vi "PathPlanner_TrajectoryState25_Interpolate.vi"(9 "Time":dbl, 10 "end Val":T1={"TimeSeconds"=0.0, "LinearVelocity"=0.0, "Heading"={"VALUE"=0.0, "COS"=1.0, "SIN"=0.0}, "Constraints"={"MaxVelocityMps;"=0.0, "MaxAccelerationMpsSq;"=0.0, "MaxAngularVelRadPsEc;"=0.0, "MaxAngularAccRadPSecSq"=0.0, "Exists"=FALSE, "Unlimited"=FALSE, "NominalVoltageVolts"=12.0}, "DeltaPos"=0.0, "FieldSpeeds"={"vX"=0.0, "vY"=0.0, "vOmega"=0.0}, "pose"={"TRANSLATION"={"X"=0.0, "Y"=0.0}, "ROTATION"={"VALUE"=0.0, "COS"=1.0, "SIN"=0.0}}, "DeltaRot"={"VALUE"=0.0, "COS"=1.0, "SIN"=0.0}, "ModuleStates"=[], "WaypointRelPos"=0.0, "Feedforwards"={"accelerationsMPSSq"=[], "linearForcesNewtons"=[], "torqueCurrentsAmps"=[], "robotRelativeForcesXNewtons"=[], "robotRelativeForcesYNewtons"=[]}} {"ModuleStates"."SWERVE_DRIVE_MODULE_STATE"."Angle"."SIN" format="%13.4f"; "ModuleStates"."SWERVE_DRIVE_MODULE_STATE"."Angle"."COS" format="%13.4f"; "ModuleStates"."SWERVE_DRIVE_MODULE_STATE"."Angle"."VALUE" format="%13.4f"; "ModuleStates"."FieldAngle"."SIN" format="%13.4f"; "ModuleStates"."FieldAngle"."COS" format="%13.4f"; "ModuleStates"."FieldAngle"."VALUE" format="%13.4f"; "ModuleStates"."FieldPos"."Y" format="%14.3f"; "ModuleStates"."FieldPos"."X" format="%14.3f"; "DeltaRot"."SIN" format="%13.4f"; "DeltaRot"."COS" format="%13.4f"; "DeltaRot"."VALUE" format="%13.4f"; "pose"."ROTATION"."SIN" format="%13.4f"; "pose"."ROTATION"."COS" format="%13.4f"; "pose"."ROTATION"."VALUE" format="%13.4f"; "pose"."TRANSLATION"."Y" format="%14.3f"; "pose"."TRANSLATION"."X" format="%14.3f"; "FieldSpeeds"."vOmega" format="%10.3f"; "FieldSpeeds"."vY" format="%10.3f"; "FieldSpeeds"."vX" format="%10.3f"; "Heading"."SIN" format="%13.4f"; "Heading"."COS" format="%13.4f"; "Heading"."VALUE" format="%13.4f"}, 11 "in PathPlannerState":T1={"TimeSeconds"=0.0, "LinearVelocity"=0.0, "Heading"={"VALUE"=0.0, "COS"=1.0, "SIN"=0.0}, "Constraints"={"MaxVelocityMps;"=0.0, "MaxAccelerationMpsSq;"=0.0, "MaxAngularVelRadPsEc;"=0.0, "MaxAngularAccRadPSecSq"=0.0, "Exists"=FALSE, "Unlimited"=FALSE, "NominalVoltageVolts"=12.0}, "DeltaPos"=0.0, "FieldSpeeds"={"vX"=0.0, "vY"=0.0, "vOmega"=0.0}, "pose"={"TRANSLATION"={"X"=0.0, "Y"=0.0}, "ROTATION"={"VALUE"=0.0, "COS"=1.0, "SIN"=0.0}}, "DeltaRot"={"VALUE"=0.0, "COS"=1.0, "SIN"=0.0}, "ModuleStates"=[], "WaypointRelPos"=0.0, "Feedforwards"={"accelerationsMPSSq"=[], "linearForcesNewtons"=[], "torqueCurrentsAmps"=[], "robotRelativeForcesXNewtons"=[], "robotRelativeForcesYNewtons"=[]}} {"ModuleStates"."SWERVE_DRIVE_MODULE_STATE"."Angle"."SIN" format="%13.4f"; "ModuleStates"."SWERVE_DRIVE_MODULE_STATE"."Angle"."COS" format="%13.4f"; "ModuleStates"."SWERVE_DRIVE_MODULE_STATE"."Angle"."VALUE" format="%13.4f"; "ModuleStates"."FieldAngle"."SIN" format="%13.4f"; "ModuleStates"."FieldAngle"."COS" format="%13.4f"; "ModuleStates"."FieldAngle"."VALUE" format="%13.4f"; "ModuleStates"."FieldPos"."Y" format="%14.3f"; "ModuleStates"."FieldPos"."X" format="%14.3f"; "DeltaRot"."SIN" format="%13.4f"; "DeltaRot"."COS" format="%13.4f"; "DeltaRot"."VALUE" format="%13.4f"; "pose"."ROTATION"."SIN" format="%13.4f"; "pose"."ROTATION"."COS" format="%13.4f"; "pose"."ROTATION"."VALUE" format="%13.4f"; "pose"."TRANSLATION"."Y" format="%14.3f"; "pose"."TRANSLATION"."X" format="%14.3f"; "FieldSpeeds"."vOmega" format="%10.3f"; "FieldSpeeds"."vY" format="%10.3f"; "FieldSpeeds"."vX" format="%10.3f"; "Heading"."SIN" format="%13.4f"; "Heading"."COS" format="%13.4f"; "Heading"."VALUE" format="%13.4f"}) -> (3 "interpolated PathPlanner State":T1={"TimeSeconds"=0.0, "LinearVelocity"=0.0, "Heading"={"VALUE"=0.0, "COS"=1.0, "SIN"=0.0}, "Constraints"={"MaxVelocityMps;"=0.0, "MaxAccelerationMpsSq;"=0.0, "MaxAngularVelRadPsEc;"=0.0, "MaxAngularAccRadPSecSq"=0.0, "Exists"=FALSE, "Unlimited"=FALSE, "NominalVoltageVolts"=12.0}, "DeltaPos"=0.0, "FieldSpeeds"={"vX"=0.0, "vY"=0.0, "vOmega"=0.0}, "pose"={"TRANSLATION"={"X"=0.0, "Y"=0.0}, "ROTATION"={"VALUE"=0.0, "COS"=1.0, "SIN"=0.0}}, "DeltaRot"={"VALUE"=0.0, "COS"=1.0, "SIN"=0.0}, "ModuleStates"=[], "WaypointRelPos"=0.0, "Feedforwards"={"accelerationsMPSSq"=[], "linearForcesNewtons"=[], "torqueCurrentsAmps"=[], "robotRelativeForcesXNewtons"=[], "robotRelativeForcesYNewtons"=[]}} {"ModuleStates"."SWERVE_DRIVE_MODULE_STATE"."Angle"."SIN" format="%13.4f"; "ModuleStates"."SWERVE_DRIVE_MODULE_STATE"."Angle"."COS" format="%13.4f"; "ModuleStates"."SWERVE_DRIVE_MODULE_STATE"."Angle"."VALUE" format="%13.4f"; "ModuleStates"."FieldAngle"."SIN" format="%13.4f"; "ModuleStates"."FieldAngle"."COS" format="%13.4f"; "ModuleStates"."FieldAngle"."VALUE" format="%13.4f"; "ModuleStates"."FieldPos"."Y" format="%14.3f"; "ModuleStates"."FieldPos"."X" format="%14.3f"; "DeltaRot"."SIN" format="%13.4f"; "DeltaRot"."COS" format="%13.4f"; "DeltaRot"."VALUE" format="%13.4f"; "pose"."ROTATION"."SIN" format="%13.4f"; "pose"."ROTATION"."COS" format="%13.4f"; "pose"."ROTATION"."VALUE" format="%13.4f"; "pose"."TRANSLATION"."Y" format="%14.3f"; "pose"."TRANSLATION"."X" format="%14.3f"; "FieldSpeeds"."vOmega" format="%10.3f"; "FieldSpeeds"."vY" format="%10.3f"; "FieldSpeeds"."vX" format="%10.3f"; "Heading"."SIN" format="%13.4f"; "Heading"."COS" format="%13.4f"; "Heading"."VALUE" format="%13.4f"})   [LabVIEW 2019, in "PathPlanner24.lvlib"]
doc: "Interpolate between this state and the given state\n \nInputs: \n - trajectoryState - cluster - this trajectory state\n - endVal - cluster - State to interpolate with\n - t - double - Interpolation factor (0.0-1.0)\n\nOutputs:\n - Interpolated state - trajectory state - interpolated state"
uses:
  PathPlanner24.lvlib
  TypeDef/PathPlannerTrajectoryState25.ctl
  <vilib>/Rock Robotics/WPI/ThirdParty/JAS_Junk/TrajLib/TypeDef/ROTATION2D.ctl
  TypeDef/PathPlannerPathConstraints.ctl
  <vilib>/Rock Robotics/WPI/ThirdParty/JAS_Junk/TrajLib/TypeDef/CHASSIS_SPEEDS.ctl
  <vilib>/Rock Robotics/WPI/ThirdParty/JAS_Junk/TrajLib/TypeDef/POSE2D.ctl
  <vilib>/Rock Robotics/WPI/ThirdParty/JAS_Junk/TrajLib/TypeDef/TRANSLATION2D.ctl
  TypeDef/PathPlannerSwerveModTrajState.ctl
  <vilib>/Rock Robotics/WPI/ThirdParty/JAS_Junk/TrajLib/TypeDef/SWERVE_DRIVE_MODULE_STATE.ctl
  TypeDef/PathPlannerDriveFeedFwds.ctl
  <vilib>/Rock Robotics/WPI/ThirdParty/JAS_Junk/TrajLib/MathUtil_Interpolate.vi
  <vilib>/Rock Robotics/WPI/ThirdParty/JAS_Junk/TrajLib/Rotation2d_Minus.vi
  <vilib>/Rock Robotics/WPI/ThirdParty/JAS_Junk/TrajLib/Rotation2d_Times.vi
  <vilib>/Rock Robotics/WPI/ThirdParty/JAS_Junk/TrajLib/Rotation2d_Plus.vi
  <vilib>/Rock Robotics/WPI/ThirdParty/JAS_Junk/TrajLib/MathUtil_Clamp.vi
  <vilib>/Rock Robotics/WPI/ThirdParty/JAS_Junk/TrajLib/Rotation2d_UnaryMinus.vi
  <vilib>/Rock Robotics/WPI/ThirdParty/JAS_Junk/TrajLib/Rotation2d_RotateBy.vi
  <vilib>/Rock Robotics/WPI/ThirdParty/JAS_Junk/TrajLib/Rotation2d_CreateAngle.vi
  <vilib>/Rock Robotics/WPI/ThirdParty/JAS_Junk/TrajLib/Rotation2d_CreateXY.vi
  <vilib>/Rock Robotics/WPI/ThirdParty/JAS_Junk/TrajLib/Util_CalcDist.vi
  <vilib>/Rock Robotics/WPI/ThirdParty/JAS_Junk/TrajLib/Trajectory_Library.lvlib
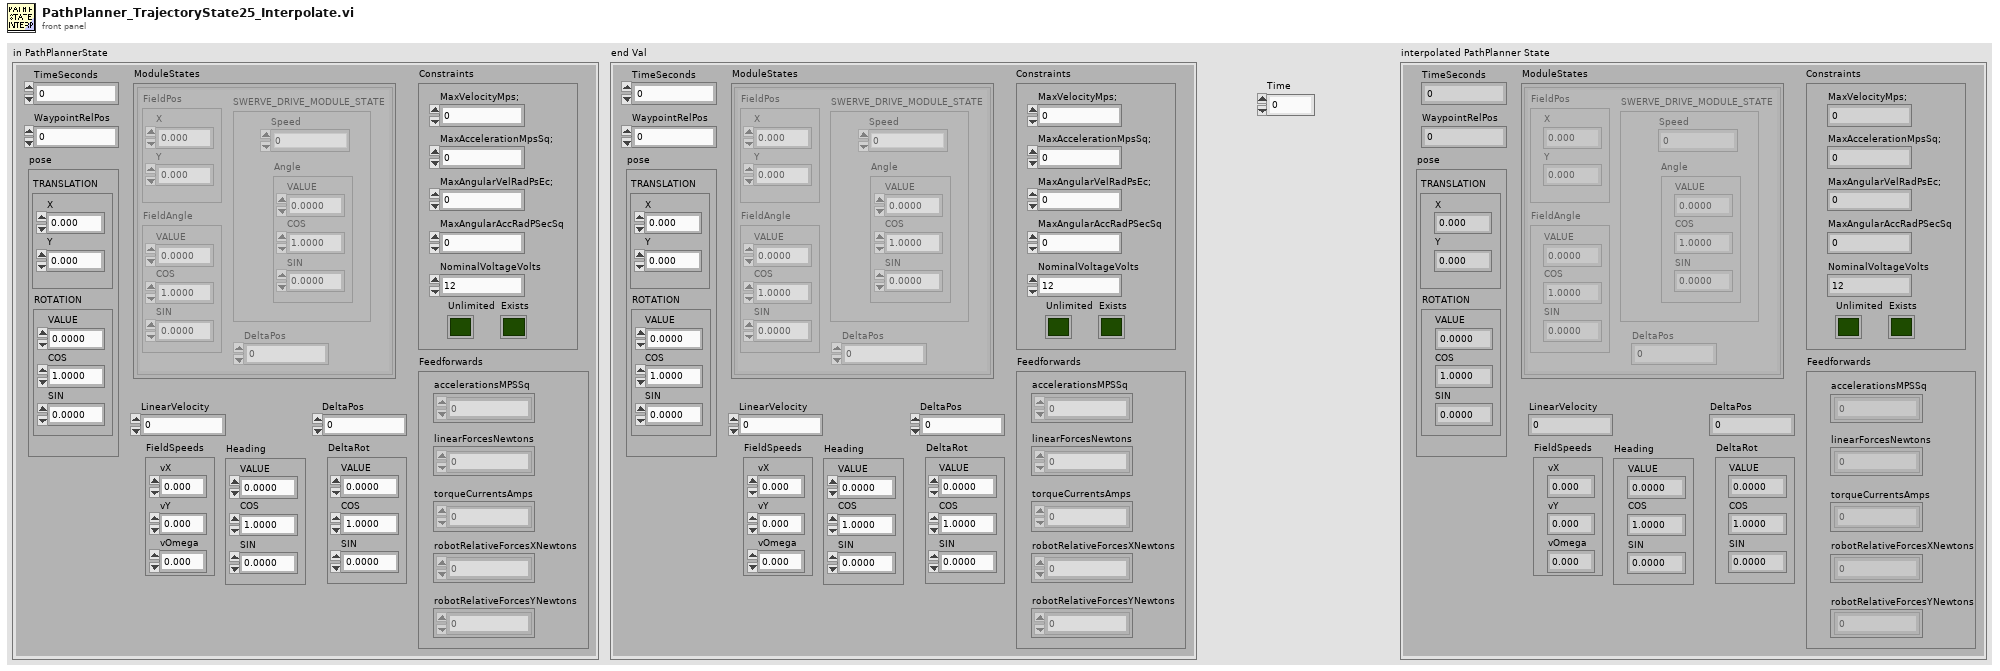
[diagram p1: front panel]
types:
  T1 = typedef "PathPlanner24.lvlib/PathPlannerTrajectoryState25.ctl" = cluster{"TimeSeconds":dbl, "LinearVelocity":dbl, "Heading":T2, "Constraints":T3, "DeltaPos":dbl, "FieldSpeeds":T4, "pose":T5, "DeltaRot":T2, "ModuleStates":T7[], "WaypointRelPos":dbl, "Feedforwards":T9}
  T2 = typedef "Trajectory_Library.lvlib/ROTATION2D.ctl" = cluster{"VALUE":dbl, "COS":dbl, "SIN":dbl}
  T3 = typedef "PathPlanner24.lvlib/PathPlannerPathConstraints.ctl" = cluster{"MaxVelocityMps;":dbl, "MaxAccelerationMpsSq;":dbl, "MaxAngularVelRadPsEc;":dbl, "MaxAngularAccRadPSecSq":dbl, "Exists":bool, "Unlimited":bool, "NominalVoltageVolts":dbl}
  T4 = typedef "Trajectory_Library.lvlib/CHASSIS_SPEEDS.ctl" = cluster{"vX":dbl, "vY":dbl, "vOmega":dbl}
  T5 = typedef "Trajectory_Library.lvlib/POSE2D.ctl" = cluster{"TRANSLATION":T6, "ROTATION":T2}
  T6 = typedef "Trajectory_Library.lvlib/TRANSLATION2D.ctl" = cluster{"X":dbl, "Y":dbl}
  T7 = typedef "PathPlanner24.lvlib/PathPlannerSwerveModTrajState.ctl" = cluster{"FieldPos":T6, "FieldAngle":T2, "DeltaPos":dbl, "SWERVE_DRIVE_MODULE_STATE":T8}
  T8 = typedef "Trajectory_Library.lvlib/SWERVE_DRIVE_MODULE_STATE.ctl" = cluster{"Speed":dbl, "Angle":T2}
  T9 = typedef "PathPlanner24.lvlib/PathPlannerDriveFeedFwds.ctl" = cluster{"accelerationsMPSSq":dbl[], "linearForcesNewtons":dbl[], "torqueCurrentsAmps":dbl[], "robotRelativeForcesXNewtons":dbl[], "robotRelativeForcesYNewtons":dbl[]}
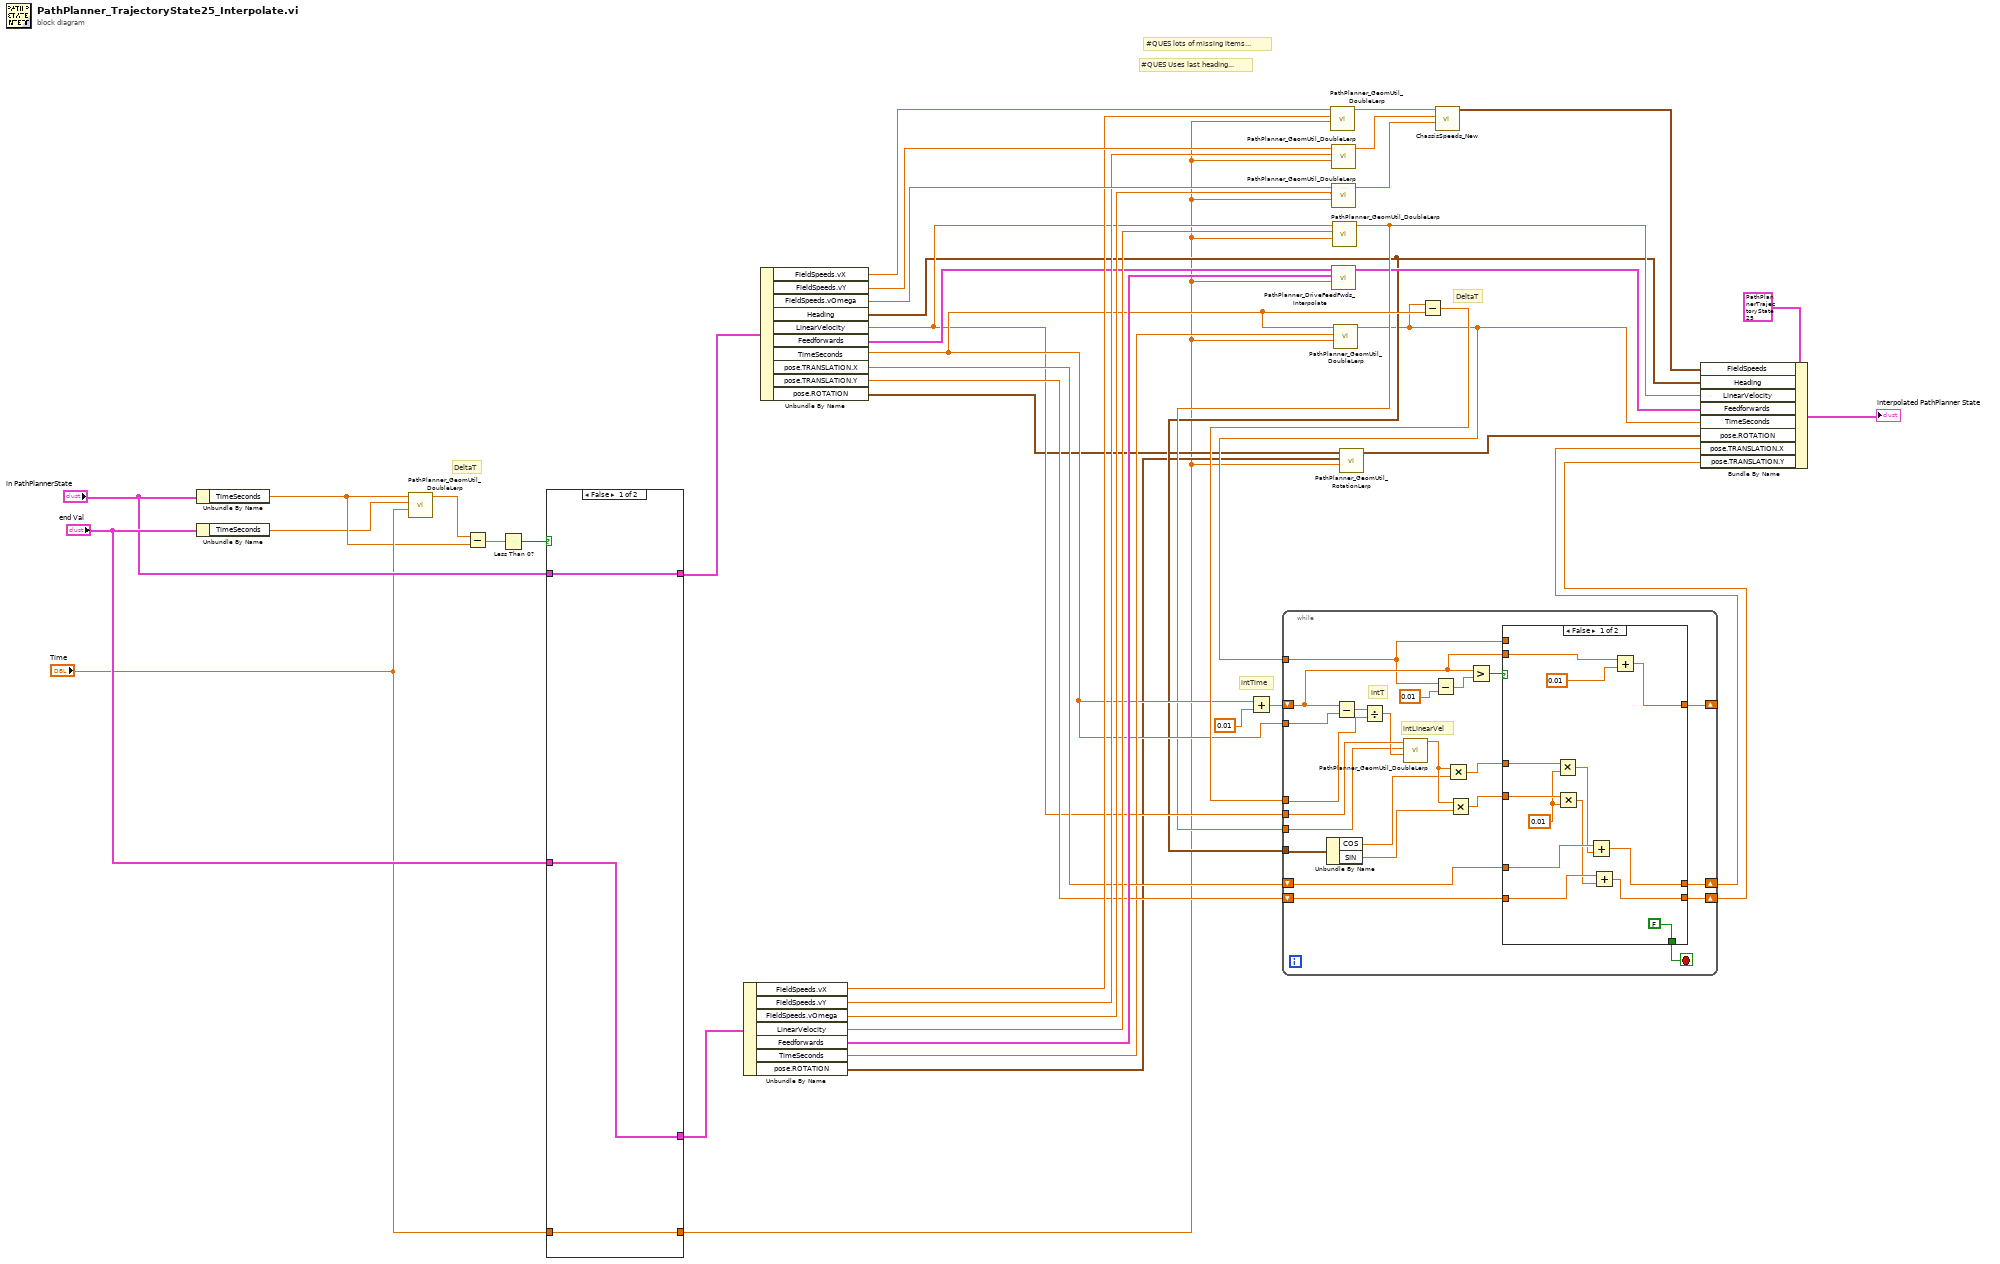
[diagram p0: block diagram]
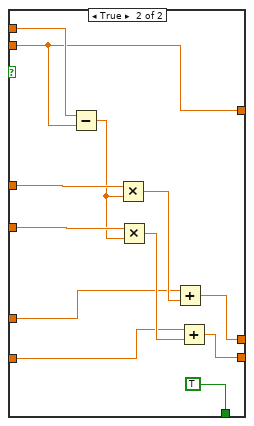
[diagram p2: hidden frame]
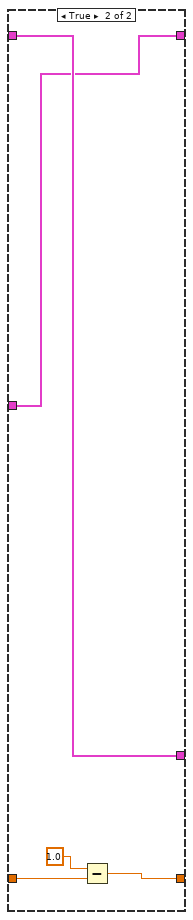
[diagram p3: hidden frame]
diagram:
  # "#QUES lots of missing items..."
  # "intTime"
  # "DeltaT"
  # "#QUES Uses last heading..."
  # "DeltaT"
  n1 = Unbundle By Name("in PathPlannerState") -> ("TimeSeconds"=w23:dbl)
  n2 = Unbundle By Name("end Val") -> ("TimeSeconds"=w22:dbl)
  n3 = call "PathPlanner_GeomUtil_DoubleLerp.vi"("T"="Time", "EndVal"=w22, "StartVal"=w23) -> ("Lerp"=w24:dbl)  [unwired: 8 in]
  n4 = Subtract(x=w24, y=w23) -> (x-y=w41:dbl)
  n5 = Less Than 0?(x=w41) -> (x < 0?=w40:bool)
  n6 = case shown="False" w40 {
    tunnel: "end Val" -> [w46 w50]
    tunnel: [w46 w51] -> w35
    tunnel: "in PathPlannerState" -> [w45 w51]
    tunnel: [w45 w50] -> w36
    tunnel: [w44 w47] -> w1
    tunnel: "Time" -> [w44 w48]
    frame False {
    }
    frame True {
      n7 = Subtract(x=1.0, y=w48) -> (x-y=w47:dbl)
    }
  }
  n8 = Unbundle By Name(w35) -> ("FieldSpeeds.vX"=w25:dbl, "FieldSpeeds.vY"=w26:dbl, "FieldSpeeds.vOmega"=w27:dbl, "LinearVelocity"=w21:dbl, "Feedforwards"=w19:T9, "TimeSeconds"=w14:dbl, "pose.ROTATION"=w5:T2)
  n9 = Unbundle By Name(w36) -> ("FieldSpeeds.vX"=w34:dbl, "FieldSpeeds.vY"=w33:dbl, "FieldSpeeds.vOmega"=w32:dbl, "Heading"=w8:T2, "LinearVelocity"=w11:dbl, "Feedforwards"=w20:T9, "TimeSeconds"=w12:dbl, "pose.TRANSLATION.X"=w16:dbl, "pose.TRANSLATION.Y"=w15:dbl, "pose.ROTATION"=w6:T2)
  n10 = Add(x=w12, y=0.01) -> (x+y=w17:dbl)
  n11 = call "PathPlanner_GeomUtil_DoubleLerp.vi"("T"=w1, "EndVal"=w25, "StartVal"=w34) -> ("Lerp"=w31:dbl)  [unwired: 8 in]
  n12 = call "PathPlanner_GeomUtil_DoubleLerp.vi"("T"=w1, "EndVal"=w26, "StartVal"=w33) -> ("Lerp"=w30:dbl)  [unwired: 8 in]
  n13 = call "PathPlanner_GeomUtil_DoubleLerp.vi"("T"=w1, "EndVal"=w27, "StartVal"=w32) -> ("Lerp"=w29:dbl)  [unwired: 8 in]
  n14 = call "PathPlanner_DriveFeedFwds_Interpolate.vi"("Time"=w1, "end Val"=w19, "in DriveFeedFwds"=w20) -> ("interpolated DriveFeedFwds"=w9:T9)  [unwired: 8 in]
  n15 = call "PathPlanner_GeomUtil_DoubleLerp.vi"("T"=w1, "EndVal"=w21, "StartVal"=w11) -> ("Lerp"=w10:dbl)  [unwired: 8 in]
  n16 = call "PathPlanner_GeomUtil_DoubleLerp.vi"("T"=w1, "EndVal"=w14, "StartVal"=w12) -> ("Lerp"=w7:dbl)  [unwired: 8 in]
  n17 = call "PathPlanner_GeomUtil_RotationLerp.vi"("T"=w1, "EndVal"=w5, "StartVal"=w6) -> ("Lerp"=w4:T2)  [unwired: 8 in]
  n18 = Subtract(x=w7, y=w12) -> (x-y=w13:dbl)
  n19 = while {
    shift-right: [w56] -> w3
    shift-left: w16 -> [w58]
    shift-right: [w55] -> w2
    shift-left: w15 -> [w57]
    shift-right: [w59] -> _
    shift-left: w17 -> [w60]
    tunnel: w13 -> [w72]
    tunnel: w12 -> [w74]
    tunnel: w11 -> [w71]
    tunnel: w10 -> [w69]
    tunnel: w8 -> [w68]
    tunnel: w7 -> [w52]
    stop <- w61 stop-if-true
    # "intLinearVel"
    # "intT"
    n20 = Unbundle By Name(w68) -> ("COS"=w66:dbl, "SIN"=w65:dbl)
    n21 = Subtract(x=w60, y=w74) -> (x-y=w73:dbl)
    n22 = Divide(x=w73, y=w72) -> (x/y=w70:dbl)
    n23 = call "PathPlanner_GeomUtil_DoubleLerp.vi"("T"=w70, "EndVal"=w69, "StartVal"=w71) -> ("Lerp"=w67:dbl)  [unwired: 8 in]
    n24 = Subtract(x=w52, y=0.01) -> (x-y=w64:dbl)
    n25 = Multiply(x=w67, y=w66) -> (x*y=w54:dbl)
    n26 = Multiply(x=w67, y=w65) -> (x*y=w53:dbl)
    n27 = Greater?(x=w60, y=w64) -> (0:w62:bool)
    n28 = case shown="False" w62 {
      tunnel: [FALSE TRUE] -> w61
      tunnel: w60 -> [w86 w95]
      tunnel: [w84 w95] -> w59
      tunnel: w58 -> [w83 w91]
      tunnel: w57 -> [w82 w90]
      tunnel: [w81 w89] -> w56
      tunnel: [w80 w88] -> w55
      tunnel: w54 -> [w79 w94]
      tunnel: w53 -> [w78 w93]
      tunnel: w52 -> [_ w96]
      frame False {
        w77 = 0.01 ("y")
        n29 = Multiply(x=w79, y=w77) -> (x*y=w76:dbl)
        n30 = Multiply(x=w78, y=w77) -> (x*y=w75:dbl)
        n31 = Add(x=w83, y=w76) -> (x+y=w81:dbl)
        n32 = Add(x=w82, y=w75) -> (x+y=w80:dbl)
        n33 = Add(x=w86, y=0.01) -> (x+y=w84:dbl)
      }
      frame True {
        n34 = Subtract(x=w96, y=w95) -> (x-y=w92:dbl)
        n35 = Multiply(x=w94, y=w92) -> (x*y=w98:dbl)
        n36 = Multiply(x=w93, y=w92) -> (x*y=w97:dbl)
        n37 = Add(x=w91, y=w98) -> (x+y=w89:dbl)
        n38 = Add(x=w90, y=w97) -> (x+y=w88:dbl)
      }
    }
  }
  n39 = call <vilib>:"ChassisSpeeds_New.vi"("vAngular"=w29, "vY"=w30, "vX"=w31) -> ("CHASSIS"=w28:T4)  [unwired: 8 in]
  n40 = Bundle By Name(cluster=T1 {"TimeSeconds"=0.0, "LinearVelocity"=0.0, "Heading"={"VALUE"=0.0, "COS"=1.0, "SIN"=0.0}, "Constraints"={"MaxVelocityMps;"=0.0, "MaxAccelerationMpsSq;"=0.0, "MaxAngularVelRadPsEc;"=0.0, "MaxAngularAccRadPSecSq"=0.0, "Exists"=FALSE, "Unlimited"=FALSE, "NominalVoltageVolts"=12.0}, "DeltaPos"=0.0, "FieldSpeeds"={"vX"=0.0, "vY"=0.0, "vOmega"=0.0}, "pose"={"TRANSLATION"={"X"=0.0, "Y"=0.0}, "ROTATION"={"VALUE"=0.0, "COS"=1.0, "SIN"=0.0}}, "DeltaRot"={"VALUE"=0.0, "COS"=1.0, "SIN"=0.0}, "ModuleStates"=[], "WaypointRelPos"=0.0, "Feedforwards"={"accelerationsMPSSq"=[], "linearForcesNewtons"=[], "torqueCurrentsAmps"=[], "robotRelativeForcesXNewtons"=[], "robotRelativeForcesYNewtons"=[]}} ("PathPlannerState"), "FieldSpeeds"=w28, "Heading"=w8, "LinearVelocity"=w10, "Feedforwards"=w9, "TimeSeconds"=w7, "pose.ROTATION"=w4, "pose.TRANSLATION.X"=w3, "pose.TRANSLATION.Y"=w2) -> (→"interpolated PathPlanner State":T1)
